vi "log analysis_gps.vi"() -> ()   [LabVIEW 2019] (continued)
status\t11.949995\t14.704483\t9.772900\t-0.969253\t0.581650\t-123.913706\t0.488000\t-0.010000\n\t\n15:53:01.0\tlog_raw\tgps_raw\t#INSPVAXA,USB3,0,51.0,FINESTEERING,2107,283999.000,02000000,471d,15824;INS_ALIGNMENT_COMPLETE,INS_RTKFIXED,37.37026095503,126.72096836486,9.7766,22.3000,-0.3661,-0.3031,0.0412,-0.630265217,0.537624421,214.046710084,0.4317,0.3034,0.5943,0.1125,0.0938,0.0813,0.0958,0.0998,5.2748,0f000001,0*95a9afe3\n\tsystem status\tnormal 2 27.800000 0 0\trobot status\t11.803932\t14.512173\t9.776600\t-0.630265\t0.537624\t-124.046710\t0.489000\t-0.001000\n\t\n15:53:01.5\tlog_raw\tgps_raw\t#INSPVAXA,USB3,0,49.5,FINESTEERING,2107,283999.500,02000000,471d,15824;INS_ALIGNMENT_COMPLETE,INS_RTKFIXED,37.37025925101,126.72096675133,9.7788,22.3000,-0.3833,-0.2925,0.0276,-0.676998170,0.665326171,214.262149706,0.4315,0.3034,0.5944,0.1124,0.0937,0.0810,0.0958,0.0998,5.2762,0f000001,0*6af82f9f\n\tsystem status\tnormal 2 27.800000 0 0\trobot status\t11.661008\t14.323053\t9.778800\t-0.676998\t0.665326\t-124.262150\t0.491000\t-0.002000\n\t\n15:53:02.0\tlog_raw\tgps_raw\t#DUALANTENNAHEADINGA,USB3,0,49.5,FINESTEERING,2107,284000.000,02000000,d426,15824;INSUFFICIENT_OBS,NONE,-1.000000000,0.000000000,0.000000000,0.0,0.000000000,0.000000000,\"631T\",10,3,3,3,04,00,20,00*77bc98b4\n\tsystem status\tnormal 2 27.800000 0 0\trobot status\t11.517592\t14.132192\t9.783800\t-0.972120\t0.567935\t-124.365534\t0.491000\t-0.010000\n\t\n15:53:02.5\tlog_raw\tgps_raw\t#INSPVAXA,USB3,0,51.5,FINESTEERING,2107,284000.500,02000000,471d,15824;INS_ALIGNMENT_COMPLETE,INS_RTKFIXED,37.37025584789,126.72096350983,9.7893,22.3000,-0.3628,-0.2938,0.0413,-0.857969709,0.678060682,214.382554495,0.4312,0.3037,0.5943,0.1122,0.0935,0.0807,0.0958,0.0998,5.2776,0f000001,0*ebd8e3c0\n\tsystem status\tnormal 2 27.800000 0 0\trobot status\t11.373882\t13.945360\t9.789300\t-0.857970\t0.678061\t-124.382554\t0.484000\t0.001000\n\t\n15:53:03.0\tlog_raw\tgps_raw\t#INSPVAXA,USB3,0,51.5,FINESTEERING,2107,284001.000,02000000,471d,15824;INS_ALIGNMENT_COMPLETE,INS_RTKFIXED,37.37025415125,126.72096186926,9.7945,22.3000,-0.3741,-0.3078,0.0321,-0.868538574,0.838914865,214.492970647,0.4312,0.3037,0.5943,0.1122,0.0935,0.0807,0.0958,0.0998,5.2776,0f000001,0*3e03e893\n\tsystem status\tnormal 2 27.800000 0 0\trobot status\t11.228563\t13.757059\t9.794500\t-0.868539\t0.838915\t-124.492971\t0.495000\t0.003000\n\t\n15:53:03.5\tlog_raw\tgps_raw\t#INSPVAXA,USB3,0,51.5,FINESTEERING,2107,284001.500,02000000,471d,15824;INS_ALIGNMENT_COMPLETE,INS_RTKFIXED,37.37025245958,126.72096024152,9.7991,22.3000,-0.3759,-0.3085,0.0182,-0.727729305,0.679989814,214.645667926,0.4313,0.3035,0.5942,0.1121,0.0935,0.0804,0.0958,0.0999,5.2791,0f000001,0*dc1168a6\n\tsystem status\tnormal 2 27.700000 0 0\trobot status\t11.084380\t13.569310\t9.799100\t-0.727729\t0.679990\t-124.645668\t0.489000\t0.000000\n\t\n15:53:04.0\tlog_raw\tgps_raw\t#INSPVAXA,USB3,0,51.5,FINESTEERING,2107,284002.000,02000000,471d,15824;INS_ALIGNMENT_COMPLETE,INS_RTKFIXED,37.37025076480,126.72095861170,9.8045,22.3000,-0.3744,-0.3095,0.0470,-0.816843186,0.787318201,214.620444446,0.4313,0.3035,0.5942,0.1121,0.0935,0.0804,0.0958,0.0999,5.2791,0f000001,0*a2e8b743\n\tsystem status\tnormal 2 27.800000 0 0\trobot status\t10.940013\t13.381215\t9.804500\t-0.816843\t0.787318\t-124.620444\t0.499000\t-0.003000\n\t\n15:53:04.5\tlog_raw\tgps_raw\t#INSPVAXA,USB3,0,51.5,FINESTEERING,2107,284002.500,02000000,471d,15824;INS_ALIGNMENT_COMPLETE,INS_RTKFIXED,37.37024907128,126.72095697824,9.8087,22.3000,-0.3691,-0.2994,0.0299,-0.885724025,0.937533929,214.679042241,0.4311,0.3036,0.5939,0.1121,0.0934,0.0802,0.0958,0.0999,5.2806,0f000001,0*c448775c\n\tsystem status\tnormal 2 27.800000 0 0\trobot status\t10.795324\t13.193261\t9.808700\t-0.885724\t0.937534\t-124.679042\t0.501000\t-0.012000\n\t\n15:53:05.0\tlog_raw\tgps_raw\t#INSPVAXA,USB3,0,51.5,FINESTEERING,2107,284003.000,02000000,471d,15824;INS_ALIGNMENT_COMPLETE,INS_RTKFIXED,37.37024737149,126.72095529976,9.8122,22.3000,-0.3776,-0.3159,0.0244,-0.547028991,0.805451972,214.632048591,0.4311,0.3036,0.5939,0.1121,0.0934,0.0802,0.0958,0.0999,5.2806,0f000001,0*63822f21\n\tsystem status\tnormal 2 27.700000 0 0\trobot status\t10.646647\t13.004611\t9.812200\t-0.547029\t0.805452\t-124.632049\t0.494000\t0.008000\n\t\n15:53:05.5\tlog_raw\tgps_raw\t#INSPVAXA,USB3,0,51.5,FINESTEERING,2107,284003.500,02000000,471d,15824;INS_ALIGNMENT_COMPLETE,INS_RTKFIXED,37.37024569352,126.72095368049,9.8164,22.3000,-0.3735,-0.3059,0.0298,-0.766116345,0.775309427,214.637421132,0.4311,0.3038,0.5936,0.1120,0.0934,0.0800,0.0957,0.0999,5.2822,0f000001,0*13581e5f\n\tsystem status\tnormal 2 27.700000 0 0\trobot status\t10.503215\t12.818382\t9.816400\t-0.766116\t0.775309\t-124.637421\t0.485000\t0.012000\n\t\n15:53:06.0\tlog_raw\tgps_raw\t#INSPVAXA,USB3,0,51.5,FINESTEERING,2107,284004.000,02000000,471d,15824;INS_ALIGNMENT_COMPLETE,INS_RTKFIXED,37.37024397579,126.72095202035,9.8197,22.3000,-0.3785,-0.3116,0.0275,-0.938815319,0.810465745,214.701472535,0.4311,0.3038,0.5936,0.1120,0.0934,0.0800,0.0957,0.0999,5.2822,0f000001,0*789baddb\n\tsystem status\tnormal 2 27.700000 0 0\trobot status\t10.356162\t12.627741\t9.819700\t-0.938815\t0.810466\t-124.701473\t0.508000\t-0.001000\n\t\n15:53:06.5\tlog_raw\tgps_raw\t#DUALANTENNAHEADINGA,USB3,0,47.5,FINESTEERING,2107,284004.500,02000000,d426,15824;INSUFFICIENT_OBS,NONE,-1.000000000,0.000000000,0.000000000,0.0,0.000000000,0.000000000,\"631T\",10,3,3,3,04,00,20,00*da91d4f3\n\tsystem status\tnormal 2 27.700000 0 0\trobot status\t10.214245\t12.441454\t9.823100\t-1.059662\t0.841985\t-124.638589\t0.494000\t0.009000\n\t\n15:53:07.0\tlog_raw\tgps_raw\t#INSPVAXA,USB3,0,47.5,FINESTEERING,2107,284005.000,02000000,471d,15824;INS_ALIGNMENT_COMPLETE,INS_RTKFIXED,37.37024061401,126.72094879160,9.8273,22.3000,-0.3519,-0.2880,0.0226,-1.106323237,0.920552674,214.656768250,0.4310,0.3041,0.5933,0.1128,0.0943,0.0811,0.0957,0.0998,5.2837,0f000001,0*6ae8f33a\n\tsystem status\tnormal 2 27.700000 0 0\trobot status\t10.070165\t12.254635\t9.827300\t-1.106323\t0.920553\t-124.656768\t0.431000\t0.090000\n\t\n15:53:07.5\tlog_raw\tgps_raw\t#DUALANTENNAHEADINGA,USB3,0,51.5,FINESTEERING,2107,284005.500,02000000,d426,15824;INSUFFICIENT_OBS,NONE,-1.000000000,0.000000000,0.000000000,0.0,0.000000000,0.000000000,\"631T\",10,3,3,3,04,00,20,00*e47d0294\n\tsystem status\tnormal 2 27.700000 0 0\trobot status\t9.926271\t12.066293\t9.829900\t-1.179806\t0.971683\t-124.561454\t0.442000\t0.087000\n\t\n15:53:08.0\tlog_raw\tgps_raw\t#DUALANTENNAHEADINGA,USB3,0,51.5,FINESTEERING,2107,284006.000,02000000,d426,15824;INSUFFICIENT_OBS,NONE,-1.000000000,0.000000000,0.000000000,0.0,0.000000000,0.000000000,\"631T\",11,3,3,3,04,00,20,00*52e49efe\n\tsystem status\tnormal 2 27.700000 0 0\trobot status\t9.781553\t11.879735\t9.833700\t-1.201114\t0.886672\t-124.479449\t0.556000\t-0.075000\n\t\n15:53:08.5\tlog_raw\tgps_raw\t#INSPVAXA,USB3,0,53.0,FINESTEERING,2107,284006.500,02000000,471d,15824;INS_ALIGNMENT_COMPLETE,INS_RTKFIXED,37.37023555537,126.72094390060,9.8375,22.3000,-0.3979,-0.3155,0.0300,-1.049604395,0.780641756,214.313549456,0.4317,0.3045,0.5932,0.1125,0.0938,0.0806,0.0956,0.0998,5.2867,0f000001,0*baf56160\n\tsystem status\tnormal 2 27.700000 0 0\trobot status\t9.636928\t11.693205\t9.837500\t-1.049604\t0.780642\t-124.313549\t0.463000\t0.071000\n\t\n15:53:09.0\tlog_raw\tgps_raw\t#DUALANTENNAHEADINGA,USB3,0,53.0,FINESTEERING,2107,284007.000,02000000,d426,15824;INSUFFICIENT_OBS,NONE,-1.000000000,0.000000000,0.000000000,0.0,0.000000000,0.000000000,\"631T\",11,3,3,3,04,00,20,00*a2cfd1a3\n\tsystem status\tnormal 2 27.700000 0 0\trobot status\t9.494443\t11.506376\t9.840200\t-1.194135\t0.885259\t-124.175019\t0.475000\t0.038000\n\t\n15:53:09.5\tlog_raw\tgps_raw\t#INSPVAXA,USB3,0,51.5,FINESTEERING,2107,284007.500,02000000,471d,15824;INS_ALIGNMENT_COMPLETE,INS_RTKFIXED,37.37023216601,126.72094065037,9.8419,22.3000,-0.3656,-0.2859,0.0240,-0.929585052,0.783187506,214.018400547,0.4319,0.3042,0.5932,0.1130,0.0943,0.0814,0.0956,0.0998,5.2881,0f000001,0*b155cbfb\n\tsystem status\tnormal 2 27.700000 0 0\trobot status\t9.349028\t11.317038\t9.841900\t-0.929585\t0.783188\t-124.018401\t0.422000\t0.097000\n\t\n15:53:10.0\tlog_raw\tgps_raw\t#INSPVAXA,USB3,0,51.5,FINESTEERING,2107,284008.000,02000000,471d,15824;INS_ALIGNMENT_COMPLETE,INS_RTKFIXED,37.37023049066,126.72093905511,9.8436,22.3000,-0.3675,-0.2972,0.0326,-1.081497544,1.069523498,213.947516981,0.4319,0.3042,0.5932,0.1130,0.0943,0.0814,0.0956,0.0998,5.2881,0f000001,0*b15b7ce2\n\tsystem status\tnormal 2 27.700000 0 0\trobot status\t9.207722\t11.131100\t9.843600\t-1.081498\t1.069523\t-123.947517\t0.463000\t0.046000\n\t\n15:53:10.5\tlog_raw\tgps_raw\t#DUALANTENNAHEADINGA,USB3,0,50.5,FINESTEERING,2107,284008.500,02000000,d426,15824;INSUFFICIENT_OBS,NONE,-1.000000000,0.000000000,0.000000000,0.0,0.000000000,0.000000000,\"631T\",10,3,3,3,04,00,20,00*59d2ef86\n\tsystem status\tnormal 2 27.700000 0 0\trobot status\t9.064066\t10.938639\t9.844000\t-1.284924\t0.732388\t-123.827216\t0.577000\t-0.144000\n\t\n15:53:11.0\tlog_raw\tgps_raw\t#INSPVAXA,USB3,0,50.5,FINESTEERING,2107,284009.000,02000000,471d,15824;INS_ALIGNMENT_COMPLETE,INS_RTKFIXED,37.37022706155,126.72093581324,9.8448,22.3000,-0.3775,-0.3022,0.0342,-1.257860345,0.478173626,213.753744794,0.4320,0.3040,0.5934,0.1130,0.0939,0.0812,0.0956,0.0998,5.2894,0f000001,0*088bd23f\n\tsystem status\tnormal 2 27.700000 0 0\trobot status\t8.920563\t10.750522\t9.844800\t-1.257860\t0.478174\t-123.753745\t0.438000\t0.083000\n\t\n15:53:11.5\tlog_raw\tgps_raw\t#DUALANTENNAHEADINGA,USB3,0,50.0,FINESTEERING,2107,284009.500,02000000,d426,15824;INSUFFICIENT_OBS,NONE,-1.000000000,0.000000000,0.000000000,0.0,0.000000000,0.000000000,\"631T\",12,3,3,3,04,00,20,00*15c40b62\n\tsystem status\tnormal 2 27.700000 0 0\trobot status\t8.780675\t10.562333\t9.847300\t-1.266879\t0.595553\t-123.600213\t0.486000\t0.056000\n\t\n15:53:12.0\tlog_raw\tgps_raw\t#DUALANTENNAHEADINGA,USB3,0,50.0,FINESTEERING,2107,284010.000,02000000,d426,15824;INSUFFICIENT_OBS,NONE,-1.000000000,0.000000000,0.000000000,0.0,0.000000000,0.000000000,\"631T\",11,3,3,3,04,00,20,00*2b190075\n\tsystem status\tnormal 2 27.700000 0 0\trobot status\t8.639554\t10.375368\t9.847500\t-1.134664\t0.760063\t-123.635228\t0.544000\t-0.097000\n\t\n15:53:12.5\tlog_raw\tgps_raw\t#DUALANTENNAHEADINGA,USB3,0,52.0,FINESTEERING,2107,284010.500,02000000,d426,15824;INSUFFICIENT_OBS,NONE,-1.000000000,0.000000000,0.000000000,0.0,0.000000000,0.000000000,\"631T\",11,3,3,3,04,00,20,00*3483bc64\n\tsystem status\tnormal 2 27.800000 0 0\trobot status\t8.496932\t10.183314\t9.847900\t-1.086478\t0.615722\t-123.692564\t0.454000\t0.035000\n\t\n15:53:13.0\tlog_raw\tgps_raw\t#DUALANTENNAHEADINGA,USB3,0,52.0,FINESTEERING,2107,284011.000,02000000,d426,15824;INSUFFICIENT_OBS,NONE,-1.000000000,0.000000000,0.000000000,0.0,0.000000000,0.000000000,\"631T\",10,3,3,3,04,00,20,00*59aa29bc\n\tsystem status\tnormal 2 27.800000 0 0\trobot status\t8.355542\t9.994278\t9.852100\t-1.105677\t0.478292\t-123.710309\t0.495000\t-0.002000\n\t\n15:53:13.5\tlog_raw\tgps_raw\t#DUALANTENNAHEADINGA,USB3,0,50.0,FINESTEERING,2107,284011.500,02000000,d426,15824;INSUFFICIENT_OBS,NONE,-1.000000000,0.000000000,0.000000000,0.0,0.000000000,0.000000000,\"631T\",10,3,3,3,04,00,20,00*463095ad\n\tsystem status\tnormal 2 27.700000 0 0\trobot status\t8.216792\t9.810188\t9.856000\t-0.910019\t0.721735\t-123.699884\t0.494000\t-0.009000\n\t\n15:53:14.0\tlog_raw\tgps_raw\t#DUALANTENNAHEADINGA,USB3,0,50.0,FINESTEERING,2107,284012.000,02000000,d426,15824;INSUFFICIENT_OBS,NONE,-1.000000000,0.000000000,0.000000000,0.0,0.000000000,0.000000000,\"631T\",11,3,3,3,04,00,20,00*f0a909c7\n\tsystem status\tnormal 2 27.700000 0 0\trobot status\t8.073331\t9.623496\t9.858000\t-0.696791\t0.799201\t-123.759361\t0.484000\t-0.006000\n\t\n15:53:14.5\tlog_raw\tgps_raw\t#INSPVAXA,USB3,0,52.0,FINESTEERING,2107,284012.500,02000000,471d,15824;INS_ALIGNMENT_COMPLETE,INS_RTKFIXED,37.37021521893,126.72092466142,9.8618,22.3000,-0.3847,-0.3021,0.0234,-0.775837810,0.832251652,213.741589159,0.4316,0.3037,0.5939,0.1121,0.0935,0.0807,0.0957,0.0997,5.2927,0f000001,0*15662a94\n\tsystem status\tnormal 2 27.700000 0 0\trobot status\t7.932753\t9.436175\t9.861800\t-0.775838\t0.832252\t-123.741589\t0.512000\t-0.002000\n\t\n15:53:15.0\tlog_raw\tgps_raw\t#DUALANTENNAHEADINGA,USB3,0,52.0,FINESTEERING,2107,284013.000,02000000,d426,15824;INSUFFICIENT_OBS,NONE,-1.000000000,0.000000000,0.000000000,0.0,0.000000000,0.000000000,\"631T\",11,3,3,3,04,00,20,00*55f8a056\n\tsystem status\tnormal 2 27.700000 0 0\trobot status\t7.792601\t9.250896\t9.867200\t-0.885484\t0.744938\t-123.777160\t0.488000\t-0.007000\n\t\n15:53:15.5\tlog_raw\tgps_raw\t#DUALANTENNAHEADINGA,USB3,0,49.0,FINESTEERING,2107,284013.500,02000000,d426,15824;INSUFFICIENT_OBS,NONE,-1.000000000,0.000000000,0.000000000,0.0,0.000000000,0.000000000,\"631T\",10,3,3,3,04,00,20,00*bcdfd03e\n\tsystem status\tnormal 2 27.800000 0 0\trobot status\t7.649789\t9.065300\t9.870300\t-0.831867\t0.889724\t-123.870763\t0.483000\t-0.003000\n\t\n15:53:16.0\tlog_raw\tgps_raw\t#DUALANTENNAHEADINGA,USB3,0,49.0,FINESTEERING,2107,284014.000,02000000,d426,15824;INSUFFICIENT_OBS,NONE,-1.000000000,0.000000000,0.000000000,0.0,0.000000000,0.000000000,\"631T\",10,3,3,3,04,00,20,00*b1b5d929\n\tsystem status\tnormal 2 27.800000 0 0\trobot status\t7.505974\t8.879613\t9.872700\t-0.869968\t0.722095\t-124.014943\t0.494000\t-0.002000\n\t\n15:53:16.5\tlog_raw\tgps_raw\t#DUALANTENNAHEADINGA,USB3,0,48.0,FINESTEERING,2107,284014.500,02000000,d426,15824;INSUFFICIENT_OBS,NONE,-1.000000000,0.000000000,0.000000000,0.0,0.000000000,0.000000000,\"631T\",11,3,3,3,04,00,20,00*d5009e8c\n\tsystem status\tnormal 2 27.700000 0 0\trobot status\t7.365474\t8.693118\t9.877900\t-1.180750\t0.637885\t-124.285873\t0.492000\t-0.013000\n\t\n15:53:17.0\tlog_raw\tgps_raw\t#INSPVAXA,USB3,0,48.0,FINESTEERING,2107,284015.000,02000000,471d,15824;INS_ALIGNMENT_COMPLETE,INS_RTKFIXED,37.37020683430,126.72091660839,9.8841,22.3000,-0.3478,-0.2798,0.0325,-1.211016237,0.525489122,214.520046866,0.4313,0.3041,0.5940,0.1119,0.0933,0.0802,0.0957,0.0997,5.2955,0f000001,0*ac9f229d\n\tsystem status\tnormal 2 27.800000 0 0\trobot status\t7.219429\t8.505611\t9.884100\t-1.211016\t0.525489\t-124.520047\t0.504000\t-0.011000\n\t\n15:53:17.5\tlog_raw\tgps_raw\t#INSPVAXA,USB3,0,50.5,FINESTEERING,2107,284015.500,02000000,471d,15824;INS_ALIGNMENT_COMPLETE,INS_RTKFIXED,37.37020518291,126.72091499411,9.8875,22.3000,-0.3472,-0.2997,0.0277,-1.071436018,0.954919930,214.713975272,0.4312,0.3037,0.5941,0.1119,0.0933,0.0800,0.0957,0.0997,5.2971,0f000001,0*82bfde41\n\tsystem status\tnormal 2 27.800000 0 0\trobot status\t7.076439\t8.322332\t9.887500\t-1.071436\t0.954920\t-124.713975\t0.492000\t-0.015000\n\t\n15:53:18.0\tlog_raw\tgps_raw\t#INSPVAXA,USB3,0,50.5,FINESTEERING,2107,284016.000,02000000,471d,15824;INS_ALIGNMENT_COMPLETE,INS_RTKFIXED,37.37020352454,126.72091333889,9.8896,22.3000,-0.3642,-0.3113,0.0147,-0.944083303,0.844230452,215.071518379,0.4312,0.3037,0.5941,0.1119,0.0933,0.0800,0.0957,0.0997,5.2971,0f000001,0*acd4ef81\n\tsystem status\tnormal 2 27.800000 0 0\trobot status\t6.929822\t8.138279\t9.889600\t-0.944083\t0.844230\t-125.071518\t0.501000\t-0.010000\n\t\n15:53:18.5\tlog_raw\tgps_raw\t#DUALANTENNAHEADINGA,USB3,0,48.0,FINESTEERING,2107,284016.500,02000000,d426,15824;INSUFFICIENT_OBS,NONE,-1.000000000,0.000000000,0.000000000,0.0,0.000000000,0.000000000,\"631T\",11,3,3,3,04,00,20,00*0eb0973e\n\tsystem status\tnormal 2 27.700000 0 0\trobot status\t6.785147\t7.958517\t9.892300\t-0.977065\t0.622221\t-125.301235\t0.489000\t-0.011000\n\t\n15:53:19.0\tlog_raw\tgps_raw\t#DUALANTENNAHEADINGA,USB3,0,48.0,FINESTEERING,2107,284017.000,02000000,d426,15824;INSUFFICIENT_OBS,NONE,-1.000000000,0.000000000,0.000000000,0.0,0.000000000,0.000000000,\"631T\",10,3,3,3,04,00,20,00*639902e6\n\tsystem status\tnormal 2 27.800000 0 0\trobot status\t6.630880\t7.772419\t9.896100\t-0.837410\t0.393821\t-125.556030\t0.492000\t-0.009000\n\t\n15:53:19.5\tlog_raw\tgps_raw\t#DUALANTENNAHEADINGA,USB3,0,46.5,FINESTEERING,2107,284017.500,02000000,d426,15824;INSUFFICIENT_OBS,NONE,-1.000000000,0.000000000,0.000000000,0.0,0.000000000,0.000000000,\"631T\",10,3,3,3,04,00,20,00*f7dfbd48\n\tsystem status\tnormal 2 27.800000 0 0\trobot status\t6.484830\t7.593109\t9.897600\t-0.749165\t0.482795\t-125.861901\t0.493000\t-0.012000\n\t\n15:53:20.0\tlog_raw\tgps_raw\t#DUALANTENNAHEADINGA,USB3,0,46.5,FINESTEERING,2107,284018.000,02000000,d426,15824;INSUFFICIENT_OBS,NONE,-1.000000000,0.000000000,0.000000000,0.0,0.000000000,0.000000000,\"631T\",10,3,3,3,04,00,20,00*22979e15\n\tsystem status\tnormal 2 27.800000 0 0\trobot status\t6.329021\t7.405649\t9.898900\t-0.654914\t0.204219\t-126.090923\t0.494000\t-0.013000\n\t\n15:53:20.5\tlog_raw\tgps_raw\t#DUALANTENNAHEADINGA,USB3,0,48.0,FINESTEERING,2107,284018.500,02000000,d426,15824;INSUFFICIENT_OBS,NONE,-1.000000000,0.000000000,0.000000000,0.0,0.000000000,0.000000000,\"631T\",11,3,3,3,04,00,20,00*6133a1e3\n\tsystem status\tnormal 2 27.800000 0 0\trobot status\t6.183361\t7.230578\t9.900600\t-0.846224\t0.355757\t-126.478921\t0.492000\t-0.011000\n\t\n15:53:21.0\tlog_raw\tgps_raw\t#DUALANTENNAHEADINGA,USB3,0,48.0,FINESTEERING,2107,284019.000,02000000,d426,15824;INSUFFICIENT_OBS,NONE,-1.000000000,0.000000000,0.000000000,0.0,0.000000000,0.000000000,\"631T\",13,3,3,3,04,00,20,00*af4cb292\n\tsystem status\tnormal 2 27.800000 0 0\trobot status\t6.029653\t7.050728\t9.904100\t-0.822893\t0.455667\t-126.815251\t0.497000\t-0.019000\n\t\n15:53:21.5\tlog_raw\tgps_raw\t#DUALANTENNAHEADINGA,USB3,0,50.0,FINESTEERING,2107,284019.500,02000000,d426,15824;INSUFFICIENT_OBS,NONE,-1.000000000,0.000000000,0.000000000,0.0,0.000000000,0.000000000,\"631T\",12,3,3,3,04,00,20,00*eaa6b916\n\tsystem status\tnormal 2 27.800000 0 0\trobot status\t5.876894\t6.877619\t9.906100\t-0.703637\t0.718812\t-127.078185\t0.495000\t-0.014000\n\t\n15:53:22.0\tlog_raw\tgps_raw\t#DUALANTENNAHEADINGA,USB3,0,50.0,FINESTEERING,2107,284020.000,02000000,d426,15824;INSUFFICIENT_OBS,NONE,-1.000000000,0.000000000,0.000000000,0.0,0.000000000,0.000000000,\"631T\",10,3,3,3,04,00,20,00*262d50f0\n\tsystem status\tnormal 2 27.700000 0 0\trobot status\t5.717326\t6.698205\t9.907600\t-0.705479\t0.569323\t-127.419721\t0.494000\t-0.006000\n\t\n15:53:22.5\tlog_raw\tgps_raw\t#DUALANTENNAHEADINGA,USB3,0,48.5,FINESTEERING,2107,284020.500,02000000,d426,15824;INSUFFICIENT_OBS,NONE,-1.000000000,0.000000000,0.000000000,0.0,0.000000000,0.000000000,\"631T\",9,3,3,3,04,00,20,00*7dfaf070\n\tsystem status\tnormal 2 27.800000 0 0\trobot status\t5.565192\t6.526220\t9.909500\t-0.633197\t0.347163\t-127.711531\t0.478000\t-0.006000\n\t\n15:53:23.0\tlog_raw\tgps_raw\t#DUALANTENNAHEADINGA,USB3,0,48.5,FINESTEERING,2107,284021.000,02000000,d426,15824;INSUFFICIENT_OBS,NONE,-1.000000000,0.000000000,0.000000000,0.0,0.000000000,0.000000000,\"631T\",9,3,3,3,04,00,20,00*66d97584\n\tsystem status\tnormal 2 27.800000 0 0\trobot status\t5.407429\t6.352014\t9.913300\t-0.598640\t0.504447\t-127.980938\t0.493000\t-0.009000\n\t\n15:53:23.5\tlog_raw\tgps_raw\t#DUALANTENNAHEADINGA,USB3,0,51.5,FINESTEERING,2107,284021.500,02000000,d426,15824;INSUFFICIENT_OBS,NONE,-1.000000000,0.000000000,0.000000000,0.0,0.000000000,0.000000000,\"631T\",10,3,3,3,04,00,20,00*add87518\n\tsystem status\tnormal 2 27.800000 0 0\trobot status\t5.252800\t6.177276\t9.915700\t-0.680126\t0.618703\t-128.224651\t0.492000\t-0.009000\n\t\n15:53:24.0\tlog_raw\tgps_raw\t#DUALANTENNAHEADINGA,USB3,0,51.5,FINESTEERING,2107,284022.000,02000000,d426,15824;INSUFFICIENT_OBS,NONE,-1.000000000,0.000000000,0.000000000,0.0,0.000000000,0.000000000,\"631T\",11,3,3,3,04,00,20,00*1b41e972\n\tsystem status\tnormal 2 27.800000 0 0\trobot status\t5.093186\t6.001905\t9.916400\t-0.708995\t0.606937\t-128.432503\t0.494000\t-0.008000\n\t\n15:53:24.5\tlog_raw\tgps_raw\t#DUALANTENNAHEADINGA,USB3,0,51.0,FINESTEERING,2107,284022.500,02000000,d426,15824;INSUFFICIENT_OBS,NONE,-1.000000000,0.000000000,0.000000000,0.0,0.000000000,0.000000000,\"631T\",11,3,3,3,04,00,20,00*99281ee7\n\tsystem status\tnormal 2 27.700000 0 0\trobot status\t4.937263\t5.826013\t9.921000\t-0.968838\t0.533093\t-128.742718\t0.499000\t-0.010000\n\t\n15:53:25.0\tlog_raw\tgps_raw\t#DUALANTENNAHEADINGA,USB3,0,51.0,FINESTEERING,2107,284023.000,02000000,d426,15824;INSUFFICIENT_OBS,NONE,-1.000000000,0.000000000,0.000000000,0.0,0.000000000,0.000000000,\"631T\",11,3,3,3,04,00,20,00*23e30b67\n\tsystem status\tnormal 2 27.800000 0 0\trobot status\t4.776899\t5.651787\t9.925100\t-0.922702\t0.489039\t-128.844545\t0.497000\t0.005000\n\t\n15:53:25.5\tlog_raw\tgps_raw\t#DUALANTENNAHEADINGA,USB3,0,48.5,FINESTEERING,2107,284023.500,02000000,d426,15824;INSUFFICIENT_OBS,NONE,-1.000000000,0.000000000,0.000000000,0.0,0.000000000,0.000000000,\"631T\",11,3,3,3,04,00,20,00*80d5b0d3\n\tsystem status\tnormal 2 27.800000 0 0\trobot status\t4.617828\t5.477866\t9.926700\t-1.089911\t0.389872\t-129.027781\t0.496000\t-0.003000\n\t\n15:53:26.0\tlog_raw\tgps_raw\t\tsystem status\tnormal 2 27.700000 0 0\trobot status\t4.455319\t5.306272\t9.929300\t-0.840464\t0.179628\t-129.323373\t0.499000\t-0.005000\n\t\n15:53:26.5\tlog_raw\tgps_raw\t\tsystem status\tnormal 2 27.700000 0 0\trobot status\t4.295549\t5.134166\t9.931100\t-0.839069\t0.087002\t-129.442348\t0.494000\t-0.003000\n\t\n15:53:27.0\tlog_raw\tgps_raw\t#DUALANTENNAHEADINGA,USB3,0,50.5,FINESTEERING,2107,284025.000,02000000,d426,15824;INSUFFICIENT_OBS,NONE,-1.000000000,0.000000000,0.000000000,0.0,0.000000000,0.000000000,\"631T\",12,3,3,3,04,00,20,00*062aa131\n\tsystem status\tnormal 2 27.700000 0 0\trobot status\t4.133271\t4.963849\t9.931400\t-0.785226\t0.157731\t-129.605955\t0.491000\t-0.010000\n\t\n15:53:27.5\tlog_raw\tgps_raw\t#DUALANTENNAHEADINGA,USB3,0,50.0,FINESTEERING,2107,284025.500,02000000,d426,15824;INSUFFICIENT_OBS,NONE,-1.000000000,0.000000000,0.000000000,0.0,0.000000000,0.000000000,\"631T\",11,3,3,3,04,00,20,00*2715d00d\n\tsystem status\tnormal 2 27.800000 0 0\trobot status\t3.966807\t4.789597\t9.930300\t-0.581097\t-0.122669\t-129.802983\t0.497000\t-0.002000\n\t\n15:53:28.0\tlog_raw\tgps_raw\t#DUALANTENNAHEADINGA,USB3,0,50.0,FINESTEERING,2107,284026.000,02000000,d426,15824;INSUFFICIENT_OBS,NONE,-1.000000000,0.000000000,0.000000000,0.0,0.000000000,0.000000000,\"631T\",11,3,3,3,04,00,20,00*466ecc3f\n\tsystem status\tnormal 2 27.800000 0 0\trobot status\t3.804554\t4.622642\t9.930400\t-0.561908\t-0.215262\t-129.932798\t0.505000\t0.000000\n\t\n15:53:28.5\tlog_raw\tgps_raw\t#DUALANTENNAHEADINGA,USB3,0,52.0,FINESTEERING,2107,284026.500,02000000,d426,15824;INSUFFICIENT_OBS,NONE,-1.000000000,0.000000000,0.000000000,0.0,0.000000000,0.000000000,\"631T\",11,3,3,3,04,00,20,00*59f4702e\n\tsystem status\tnormal 2 27.800000 0 0\trobot status\t3.638219\t4.447897\t9.929600\t-0.360942\t-0.713993\t-130.170780\t0.492000\t-0.013000\n\t\n15:53:29.0\tlog_raw\tgps_raw\t#DUALANTENNAHEADINGA,USB3,0,52.0,FINESTEERING,2107,284027.000,02000000,d426,15824;INSUFFICIENT_OBS,NONE,-1.000000000,0.000000000,0.000000000,0.0,0.000000000,0.000000000,\"631T\",11,3,3,3,04,00,20,00*e33f65ae\n\tsystem status\tnormal 2 27.800000 0 0\trobot status\t3.476772\t4.280988\t9.928100\t-0.420474\t-0.472161\t-130.387582\t0.486000\t-0.012000\n\t\n15:53:29.5\tlog_raw\tgps_raw\t#DUALANTENNAHEADINGA,USB3,0,51.0,FINESTEERING,2107,284027.500,02000000,d426,15824;INSUFFICIENT_OBS,NONE,-1.000000000,0.000000000,0.000000000,0.0,0.000000000,0.000000000,\"631T\",11,3,3,3,04,00,20,00*98e10f1b\n\tsystem status\tnormal 2 27.800000 0 0\trobot status\t3.311819\t4.107458\t9.929300\t-0.536290\t-0.477111\t-130.634429\t0.498000\t-0.007000\n\t\n15:53:30.0\tlog_raw\tgps_raw\t#DUALANTENNAHEADINGA,USB3,0,51.0,FINESTEERING,2107,284028.000,02000000,d426,15824;INSUFFICIENT_OBS,NONE,-1.000000000,0.000000000,0.000000000,0.0,0.000000000,0.000000000,\"631T\",12,3,3,3,04,00,20,00*eeffaaef\n\tsystem status\tnormal 2 27.800000 0 0\trobot status\t3.146279\t3.940333\t9.927600\t-0.467007\t-0.378598\t-130.887345\t0.488000\t-0.004000\n\t\n15:53:30.5\tlog_raw\tgps_raw\t#INSPVAXA,USB3,0,53.0,FINESTEERING,2107,284028.500,02000000,471d,15824;INS_ALIGNMENT_COMPLETE,INS_RTKFIXED,37.37016418129,126.72086876057,9.9277,22.3000,-0.3056,-0.3533,0.0249,-0.407357683,-0.326305353,221.094375999,0.4345,0.3056,0.5971,0.1128,0.0942,0.0822,0.0958,0.1003,5.3097,0f000001,0*9e144474\n\tsystem status\tnormal 2 27.800000 0 0\trobot status\t2.981147\t3.771786\t9.927700\t-0.407358\t-0.326305\t-131.094376\t0.498000\t-0.010000\n\t\n15:53:31.0\tlog_raw\tgps_raw\t#DUALANTENNAHEADINGA,USB3,0,53.0,FINESTEERING,2107,284029.000,02000000,d426,15824;INSUFFICIENT_OBS,NONE,-1.000000000,0.000000000,0.000000000,0.0,0.000000000,0.000000000,\"631T\",11,3,3,3,04,00,20,00*e8f885d7\n\tsystem status\tnormal 2 27.800000 0 0\trobot status\t2.810938\t3.604038\t9.927000\t-0.204581\t-0.357296\t-131.370712\t0.495000\t-0.011000\n\t\n15:53:31.5\tlog_raw\tgps_raw\t#DUALANTENNAHEADINGA,USB3,0,48.5,FINESTEERING,2107,284029.500,02000000,d426,15824;INSUFFICIENT_OBS,NONE,-1.000000000,0.000000000,0.000000000,0.0,0.000000000,0.000000000,\"631T\",11,3,3,3,04,00,20,00*8347932b\n\tsystem status\tnormal 2 27.800000 0 0\trobot status\t2.645833\t3.436283\t9.925800\t-0.526731\t-0.296386\t-131.623611\t0.497000\t-0.008000\n\t\n15:53:32.0\tlog_raw\tgps_raw\t#DUALANTENNAHEADINGA,USB3,0,48.5,FINESTEERING,2107,284030.000,02000000,d426,15824;INSUFFICIENT_OBS,NONE,-1.000000000,0.000000000,0.000000000,0.0,0.000000000,0.000000000,\"631T\",13,3,3,3,04,00,20,00*6a781864\n\tsystem status\tnormal 2 27.800000 0 0\trobot status\t2.477724\t3.272152\t9.925900\t-0.592082\t-0.548833\t-131.830771\t0.491000\t-0.005000\n\t\n15:53:32.5\tlog_raw\tgps_raw\t#DUALANTENNAHEADINGA,USB3,0,50.0,FINESTEERING,2107,284030.500,02000000,d426,15824;INSUFFICIENT_OBS,NONE,-1.000000000,0.000000000,0.000000000,0.0,0.000000000,0.000000000,\"631T\",15,3,3,3,04,00,20,00*30d67e67\n\tsystem status\tnormal 2 27.800000 0 0\trobot status\t2.306519\t3.102203\t9.925500\t-0.607610\t-0.465484\t-132.180965\t0.490000\t-0.007000\n\t\n15:53:33.0\tlog_raw\tgps_raw\t#DUALANTENNAHEADINGA,USB3,0,50.0,FINESTEERING,2107,284031.000,02000000,d426,15824;INSUFFICIENT_OBS,NONE,-1.000000000,0.000000000,0.000000000,0.0,0.000000000,0.000000000,\"631T\",14,3,3,3,04,00,20,00*5dffebbf\n\tsystem status\tnormal 2 27.800000 0 0\trobot status\t2.136471\t2.937213\t9.924700\t-0.815122\t-0.421198\t-132.392960\t0.495000\t-0.004000\n\t\n15:53:33.5\tlog_raw\tgps_raw\t#DUALANTENNAHEADINGA,USB3,0,46.0,FINESTEERING,2107,284031.500,02000000,d426,15824;INSUFFICIENT_OBS,NONE,-1.000000000,0.000000000,0.000000000,0.0,0.000000000,0.000000000,\"631T\",14,3,3,3,04,00,20,00*d9d82858\n\tsystem status\tnormal 2 27.800000 0 0\trobot status\t1.965487\t2.771339\t9.922400\t-0.793217\t-0.473523\t-132.484141\t0.498000\t0.001000\n\t\n15:53:34.0\tlog_raw\tgps_raw\t#DUALANTENNAHEADINGA,USB3,0,46.0,FINESTEERING,2107,284032.000,02000000,d426,15824;INSUFFICIENT_OBS,NONE,-1.000000000,0.000000000,0.000000000,0.0,0.000000000,0.000000000,\"631T\",15,3,3,3,04,00,20,00*6f41b432\n\tsystem status\tnormal 2 27.800000 0 0\trobot status\t1.791892\t2.607613\t9.921700\t-0.842954\t-0.783861\t-132.863144\t0.498000\t-0.016000\n\t\n15:53:34.5\tlog_raw\tgps_raw\t#INSPVAXA,USB3,0,49.0,FINESTEERING,2107,284032.550,02000000,471d,15824;INS_ALIGNMENT_COMPLETE,INS_RTKFIXED,37.37015203193,126.72085320398,9.9212,22.3000,-0.2929,-0.3693,0.0073,-0.969546435,-0.769890504,222.991083315,0.4327,0.3047,0.5976,0.1132,0.0946,0.0822,0.0960,0.1005,5.3138,0f000001,0*7ab4b638\n\tsystem status\tnormal 2 27.800000 0 0\trobot status\t1.603170\t2.423395\t9.921200\t-0.969546\t-0.769891\t-132.991083\t0.491000\t0.001000\n\t\n15:53:35.0\tlog_raw\tgps_raw\t#INSPVAXA,USB3,0,49.0,FINESTEERING,2107,284033.050,02000000,471d,15824;INS_ALIGNMENT_COMPLETE,INS_RTKFIXED,37.37015056233,126.72085129060,9.9204,22.3000,-0.2846,-0.3575,0.0263,-1.291425678,-0.544067497,223.276181185,0.4326,0.3039,0.5975,0.1132,0.0942,0.0818,0.0959,0.1005,5.3153,0f000001,0*1faf9100\n\tsystem status\tnormal 2 27.800000 0 0\trobot status\t1.433686\t2.260292\t9.920400\t-1.291426\t-0.544067\t-133.276181\t0.493000\t-0.005000\n\t\n15:53:35.5\tlog_raw\tgps_raw\t#INSPVAXA,USB3,0,49.5,FINESTEERING,2107,284033.550,02000000,471d,15824;INS_ALIGNMENT_COMPLETE,INS_RTKFIXED,37.37014911453,126.72084937010,9.9197,22.3000,-0.2886,-0.3722,0.0073,-1.220668676,-0.203530913,223.385400784,0.4326,0.3039,0.5975,0.1132,0.0942,0.0818,0.0959,0.1005,5.3153,0f000001,0*08db545a\n\tsystem status\tnormal 2 27.800000 0 0\trobot status\t1.263571\t2.099609\t9.919700\t-1.220669\t-0.203531\t-133.385401\t0.493000\t-0.007000\n\t\n15:53:36.0\tlog_raw\tgps_raw\t\tsystem status\tnormal 2 27.800000 0 0\trobot status\t1.107191\t1.953742\t9.919200\t-1.375223\t-0.395936\t-133.526243\t0.505000\t0.006000\n\t\n15:53:36.5\tlog_raw\tgps_raw\t#DUALANTENNAHEADINGA,USB3,0,53.5,FINESTEERING,2107,284034.500,02000000,d426,15824;INSUFFICIENT_OBS,NONE,-1.000000000,0.000000000,0.000000000,0.0,0.000000000,0.000000000,\"631T\",13,3,3,3,04,00,20,00*38acfd71\n\tsystem status\tnormal 2 27.800000 0 0\trobot status\t0.935602\t1.790820\t9.918200\t-1.625962\t-0.438619\t-133.810858\t0.497000\t-0.011000\n\t\n15:53:37.0\tlog_raw\tgps_raw\t#DUALANTENNAHEADINGA,USB3,0,53.5,FINESTEERING,2107,284035.000,02000000,d426,15824;INSUFFICIENT_OBS,NONE,-1.000000000,0.000000000,0.000000000,0.0,0.000000000,0.000000000,\"631T\",13,3,3,3,04,00,20,00*8267e8f1\n\tsystem status\tnormal 2 27.800000 0 0\trobot status\t0.758933\t1.629771\t9.919000\t-1.564520\t-0.525456\t-134.046563\t0.496000\t-0.016000\n\t\n15:53:37.5\tlog_raw\tgps_raw\t#DUALANTENNAHEADINGA,USB3,0,48.5,FINESTEERING,2107,284035.500,02000000,d426,15824;INSUFFICIENT_OBS,NONE,-1.000000000,0.000000000,0.000000000,0.0,0.000000000,0.000000000,\"631T\",12,3,3,3,04,00,20,00*6b409899\n\tsystem status\tnormal 2 27.800000 0 0\trobot status\t0.587495\t1.470373\t9.918500\t-1.489483\t-0.140794\t-134.166233\t0.496000\t-0.006000\n\t\n15:53:38.0\tlog_raw\tgps_raw\t#INSPVAXA,USB3,0,48.5,FINESTEERING,2107,284036.050,02000000,471d,15824;INS_ALIGNMENT_COMPLETE,INS_RTKFIXED,37.37014185776,126.72083957018,9.9201,22.3000,-0.2874,-0.3754,0.0180,-1.581713384,-0.281316451,224.309302807,0.4333,0.3030,0.5980,0.1134,0.0944,0.0817,0.0958,0.1004,5.3150,0f000001,0*fb9a3949\n\tsystem status\tnormal 2 27.700000 0 0\trobot status\t0.395510\t1.294219\t9.920100\t-1.581713\t-0.281316\t-134.309303\t0.485000\t-0.006000\n\t\n15:53:38.5\tlog_raw\tgps_raw\t\tsystem status\tnormal 2 27.800000 0 0\trobot status\t0.237994\t1.149966\t9.919000\t-1.418153\t-0.166584\t-134.418567\t0.499000\t0.001000\n\t\n15:53:39.0\tlog_raw\tgps_raw\t#DUALANTENNAHEADINGA,USB3,0,49.0,FINESTEERING,2107,284037.000,02000000,d426,15824;INSUFFICIENT_OBS,NONE,-1.000000000,0.000000000,0.000000000,0.0,0.000000000,0.000000000,\"631T\",12,3,3,3,04,00,20,00*56ddb01a\n\tsystem status\tnormal 2 27.800000 0 0\trobot status\t0.061157\t0.990111\t9.919000\t-1.455033\t-0.247131\t-134.542724\t0.497000\t-0.010000\n\t\n15:53:39.5\tlog_raw\tgps_raw\t\tsystem status\tnormal 2 27.800000 0 0\trobot status\t-0.113601\t0.830375\t9.917900\t-1.500243\t-0.257038\t-134.656237\t0.484000\t0.003000\n\t\n15:53:40.0\tlog_raw\tgps_raw\t#DUALANTENNAHEADINGA,USB3,0,50.5,FINESTEERING,2107,284038.000,02000000,d426,15824;INSUFFICIENT_OBS,NONE,-1.000000000,0.000000000,0.000000000,0.0,0.000000000,0.000000000,\"631T\",12,3,3,3,04,00,20,00*20a328f3\n\tsystem status\tnormal 2 27.700000 0 0\trobot status\t-0.293472\t0.670709\t9.919100\t-1.309074\t-0.091552\t-134.643307\t0.501000\t0.001000\n\t\n15:53:40.5\tlog_raw\tgps_raw\t#INSPVAXA,USB3,0,49.0,FINESTEERING,2107,284038.550,02000000,471d,15824;INS_ALIGNMENT_COMPLETE,INS_RTKFIXED,37.37013464151,126.72082964109,9.9222,22.3000,-0.2992,-0.3861,0.0057,-1.451445202,0.305563653,224.751611567,0.4334,0.3031,0.5974,0.1129,0.0939,0.0810,0.0957,0.1002,5.3127,0f000001,0*124febdb\n\tsystem status\tnormal 2 27.800000 0 0\trobot status\t-0.483992\t0.493326\t9.922200\t-1.451445\t0.305564\t-134.751612\t0.499000\t0.008000\n\t\n15:53:41.0\tlog_raw\tgps_raw\t#DUALANTENNAHEADINGA,USB3,0,49.0,FINESTEERING,2107,284039.000,02000000,d426,15824;INSUFFICIENT_OBS,NONE,-1.000000000,0.000000000,0.000000000,0.0,0.000000000,0.000000000,\"631T\",12,3,3,3,04,00,20,00*395e86c7\n\tsystem status\tnormal 2 27.800000 0 0\trobot status\t-0.642074\t0.346956\t9.923100\t-1.624940\t0.464357\t-134.602298\t0.414000\t0.114000\n\t\n15:53:41.5\tlog_raw\tgps_raw\t#INSPVAXA,USB3,0,52.5,FINESTEERING,2107,284039.550,02000000,471d,15824;INS_ALIGNMENT_COMPLETE,INS_RTKFIXED,37.37013171453,126.72082571208,9.9282,22.3000,-0.2895,-0.3679,0.0213,-1.368726775,0.328135846,224.170943357,0.4333,0.3035,0.5969,0.1130,0.0937,0.0807,0.0957,0.1001,5.3122,0f000001,0*6a698e8e\n\tsystem status\tnormal 2 27.700000 0 0\trobot status\t-0.832017\t0.168477\t9.928200\t-1.368727\t0.328136\t-134.170943\t0.461000\t0.076000\n\t\n15:53:42.0\tlog_raw\tgps_raw\t#DUALANTENNAHEADINGA,USB3,0,52.5,FINESTEERING,2107,284040.000,02000000,d426,15824;INSUFFICIENT_OBS,NONE,-1.000000000,0.000000000,0.000000000,0.0,0.000000000,0.000000000,\"631T\",12,3,3,3,04,00,20,00*a1b6ba7e\n\tsystem status\tnormal 2 27.700000 0 0\trobot status\t-0.990683\t0.016167\t9.931700\t-1.360164\t0.158105\t-133.614865\t0.507000\t0.043000\n\t\n15:53:42.5\tlog_raw\tgps_raw\t#DUALANTENNAHEADINGA,USB3,0,51.5,FINESTEERING,2107,284040.500,02000000,d426,15824;INSUFFICIENT_OBS,NONE,-1.000000000,0.000000000,0.000000000,0.0,0.000000000,0.000000000,\"631T\",13,3,3,3,04,00,20,00*0d8a5093\n\tsystem status\tnormal 2 27.500000 0 0\trobot status\t-1.160197\t-0.149641\t9.932700\t-1.341061\t-0.195405\t-132.575733\t0.577000\t-0.054000\n\t\n15:53:43.0\tlog_raw\tgps_raw\t#INSPVAXA,USB3,0,49.5,FINESTEERING,2107,284041.050,02000000,471d,15824;INS_ALIGNMENT_COMPLETE,INS_RTKFIXED,37.37012716980,126.72082004347,9.9321,22.3000,-0.3311,-0.3541,0.0307,-1.568797155,-0.218407470,219.720707571,0.4330,0.3038,0.5962,0.1133,0.0947,0.0815,0.0956,0.0999,5.3092,0f000001,0*1a0eaafc\n\tsystem status\tnormal 2 27.100000 0 0\trobot status\t-1.334134\t-0.335918\t9.932100\t-1.568797\t-0.218407\t-129.720708\t0.489000\t0.167000\n\t\n15:53:43.5\tlog_raw\tgps_raw\t\tsystem status\tnormal 2 27.100000 0 0\trobot status\t-1.467886\t-0.498566\t9.931500\t-1.189903\t-0.651561\t-125.749896\t0.471000\t0.194000\n\t\n15:53:44.0\tlog_raw\tgps_raw\t#DUALANTENNAHEADINGA,USB3,0,49.5,FINESTEERING,2107,284042.000,02000000,d426,15824;INSUFFICIENT_OBS,NONE,-1.000000000,0.000000000,0.000000000,0.0,0.000000000,0.000000000,\"631T\",11,3,3,3,04,00,20,00*3086d40c\n\tsystem status\tnormal 2 27.200000 4 0\trobot status\t-1.582398\t-0.653376\t9.929400\t-1.298487\t-0.701557\t-120.235933\t0.252000\t0.202000\n\t\n15:53:44.5\tlog_raw\tgps_raw\t#INSPVAXA,USB3,0,48.5,FINESTEERING,2107,284042.550,02000000,471d,15824;INS_ALIGNMENT_COMPLETE,INS_RTKFIXED,37.37012309586,126.72081639468,9.9287,22.3000,-0.2297,-0.1271,0.0043,-1.454240344,-0.869420112,204.842413707,0.4327,0.3036,0.5960,0.1151,0.0944,0.0812,0.0955,0.0998,5.3038,0f000001,0*d43454d1\n\tsystem status\tnormal 2 27.100000 0 0\trobot status\t-1.657337\t-0.788063\t9.928700\t-1.454240\t-0.869420\t-114.842414\t0.312000\t0.169000\n\t\n15:53:45.0\tlog_raw\tgps_raw\t\tsystem status\tnormal 2 27.100000 0 0\trobot status\t-1.713359\t-0.902861\t9.927700\t-1.473849\t-0.917791\t-109.954324\t0.328000\t0.149000\n\t\n15:53:45.5\tlog_raw\tgps_raw\t\tsystem status\tnormal 2 27.100000 4 0\trobot status\t-1.760519\t-1.041247\t9.923900\t-1.436815\t-0.953248\t-104.975044\t0.281000\t0.182000\n\t\n15:53:46.0\tlog_raw\tgps_raw\t#DUALANTENNAHEADINGA,USB3,0,50.0,FINESTEERING,2107,284044.000,02000000,d426,15824;INSUFFICIENT_OBS,NONE,-1.000000000,0.000000000,0.000000000,0.0,0.000000000,0.000000000,\"631T\",10,3,3,3,04,00,20,00*24e0e22e\n\tsystem status\tnormal 2 27.100000 4 0\trobot status\t-1.798064\t-1.175012\t9.921600\t-1.333778\t-0.917194\t-99.792638\t0.329000\t0.145000\n\t\n15:53:46.5\tlog_raw\tgps_raw\t\tsystem status\tnormal 2 27.000000 4 0\trobot status\t-1.822805\t-1.316448\t9.919600\t-1.363412\t-0.950030\t-94.436758\t0.300000\t0.226000\n\t\n15:53:47.0\tlog_raw\tgps_raw\t#INSPVAXA,USB3,0,48.5,FINESTEERING,2107,284045.050,02000000,471d,15824;INS_ALIGNMENT_COMPLETE,INS_RTKFIXED,37.37011692256,126.72081439819,9.9167,22.3000,-0.2491,-0.0343,-0.0078,-1.423202522,-1.142665090,179.061069069,0.4321,0.3052,0.5955,0.1145,0.0942,0.0804,0.0954,0.0993,5.2602,0f000001,0*4754f5d4\n\tsystem status\tnormal 2 27.100000 4 0\trobot status\t-1.834183\t-1.473204\t9.916700\t-1.423203\t-1.142665\t-89.061069\t0.308000\t0.175000\n\t\n15:53:47.5\tlog_raw\tgps_raw\t#INSPVAXA,USB3,0,52.0,FINESTEERING,2107,284045.550,02000000,471d,15824;INS_ALIGNMENT_COMPLETE,INS_RTKFIXED,37.37011564365,126.72081436501,9.9153,22.3000,-0.2694,0.0262,0.0028,-1.152838671,-0.998441499,173.727062004,0.4321,0.3052,0.5955,0.1145,0.0942,0.0804,0.0954,0.0993,5.2602,0f000001,0*22f8d84c\n\tsystem status\tnormal 2 27.000000 4 0\trobot status\t-1.837122\t-1.615143\t9.915300\t-1.152839\t-0.998441\t-83.727062\t0.283000\t0.239000\n\t\n15:53:48.0\tlog_raw\tgps_raw\t#DUALANTENNAHEADINGA,USB3,0,52.0,FINESTEERING,2107,284046.000,02000000,d426,15824;INSUFFICIENT_OBS,NONE,-1.000000000,0.000000000,0.000000000,0.0,0.000000000,0.000000000,\"631T\",11,3,3,3,04,00,20,00*e03bc68c\n\tsystem status\tnormal 2 27.000000 4 0\trobot status\t-1.823175\t-1.741822\t9.914300\t-1.150899\t-0.932893\t-79.238883\t0.313000\t0.187000\n\t\n15:53:48.5\tlog_raw\tgps_raw\t#INSPVAXA,USB3,0,51.0,FINESTEERING,2107,284046.550,02000000,471d,15824;INS_ALIGNMENT_COMPLETE,INS_RTKFIXED,37.37011307842,126.72081488040,9.9123,22.3000,-0.2496,0.0473,0.0011,-1.038780714,-0.928259537,163.465097111,0.4314,0.3044,0.5952,0.1141,0.0948,0.0802,0.0953,0.0991,5.2403,0f000001,0*99f045b6\n\tsystem status\tnormal 2 27.000000 4 0\trobot status\t-1.791470\t-1.899844\t9.912300\t-1.038781\t-0.928260\t-73.465097\t0.277000\t0.204000\n\t\n15:53:49.0\tlog_raw\tgps_raw\t#INSPVAXA,USB3,0,51.0,FINESTEERING,2107,284047.050,02000000,471d,15824;INS_ALIGNMENT_COMPLETE,INS_RTKFIXED,37.37011184110,126.72081538854,9.9110,22.3000,-0.2193,0.0992,-0.0077,-0.985316738,-1.067024719,158.394367394,0.4310,0.3038,0.5948,0.1149,0.0957,0.0800,0.0951,0.0989,5.2224,0f000001,0*e0578a7c\n\tsystem status\tnormal 2 27.000000 4 0\trobot status\t-1.746460\t-2.037168\t9.911000\t-0.985317\t-1.067025\t-68.394367\t0.297000\t0.151000\n\t\n15:53:49.5\tlog_raw\tgps_raw\t#INSPVAXA,USB3,0,51.5,FINESTEERING,2107,284047.550,02000000,471d,15824;INS_ALIGNMENT_COMPLETE,INS_RTKFIXED,37.37011062254,126.72081597469,9.9105,22.3000,-0.2405,0.0932,0.0076,-1.129336312,-1.227184174,152.839130107,0.4310,0.3038,0.5948,0.1149,0.0957,0.0800,0.0951,0.0989,5.2224,0f000001,0*808c7198\n\tsystem status\tnormal 2 27.100000 4 0\trobot status\t-1.694539\t-2.172409\t9.910500\t-1.129336\t-1.227184\t-62.839130\t0.299000\t0.172000\n\t\n15:53:50.0\tlog_raw\tgps_raw\t#DUALANTENNAHEADINGA,USB3,0,51.5,FINESTEERING,2107,284048.000,02000000,d426,15824;INSUFFICIENT_OBS,NONE,-1.000000000,0.000000000,0.000000000,0.0,0.000000000,0.000000000,\"631T\",10,3,3,3,04,00,20,00*a1eded29\n\tsystem status\tnormal 2 26.900000 4 0\trobot status\t-1.633662\t-2.287353\t9.909900\t-1.039183\t-1.374027\t-58.329222\t0.287000\t0.276000\n\t\n15:53:50.5\tlog_raw\tgps_raw\t#INSPVAXA,USB3,0,51.5,FINESTEERING,2107,284048.550,02008000,471d,15824;INS_ALIGNMENT_COMPLETE,INS_RTKFIXED,37.37010828032,126.72081752863,9.9063,22.3000,-0.2254,0.1193,0.0027,-0.673231023,-1.787802383,142.480422614,0.4310,0.3033,0.5944,0.1159,0.0969,0.0798,0.0949,0.0986,5.2063,0f000001,0*d0854b13\n\tsystem status\tnormal 2 27.100000 4 0\trobot status\t-1.556894\t-2.432360\t9.906300\t-0.673231\t-1.787802\t-52.480423\t0.312000\t0.186000\n\t\n15:53:51.0\tlog_raw\tgps_raw\t#INSPVAXA,USB3,0,49.0,FINESTEERING,2107,284049.050,02008000,471d,15824;INS_ALIGNMENT_COMPLETE,INS_RTKFIXED,37.37010717885,126.72081846735,9.9026,22.3000,-0.2042,0.1830,0.0048,-0.433320353,-1.747334753,137.205490364,0.4329,0.3030,0.5941,0.1170,0.0985,0.0797,0.0945,0.0983,5.1926,0f000001,0*334c1376\n\tsystem status\t
